vi "AlliGator Create New Empty Phasor Plot.vi"(8 "Error In":errorcluster, 11 "Phasor Graph Ref":refnum<vi>) -> (0 "Error Out":errorcluster, 1 "Plot Name":string, 2 "Plot Array out":cluster{"X Array":dbl[], "Y Array":dbl[]}[](array[cluster]), 3 "Phasor Graph Ref (dup)":refnum<vi>)   [LabVIEW 2021, in "AlliGator Phasor Graph.lvlib"]
doc: "Creates empty plot in the Phasor Graph."
uses:
  <vilib>/Utility/error.llb/Error Cluster From Error Code.vi
  <vilib>/ErrorRing/Error Ring.xnode
  AlliGator Phasor Graph.lvlib
  Graphs/XY Graph/XY Graph Add-Ons.lvlib
panel:
  # "see the AlliGator License on the block diagram (Ctrl+E or Window:Show Block Diagram)"
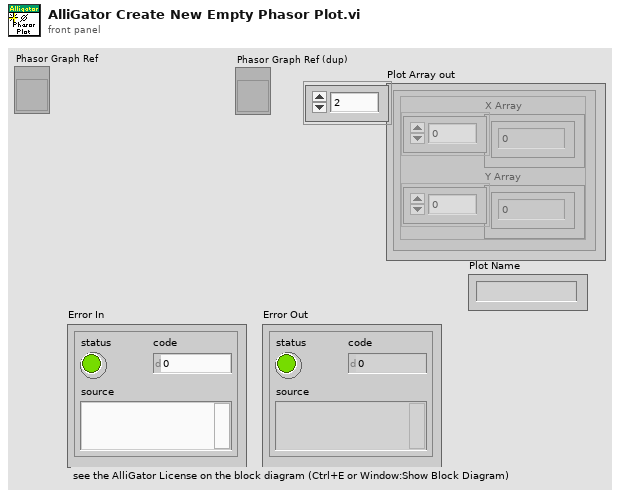
[diagram p1: front panel]
types:
  T1 = typedef "XY Graph Add-Ons.lvlib/XY Graph Refnum.ctl" = refnum<vi>
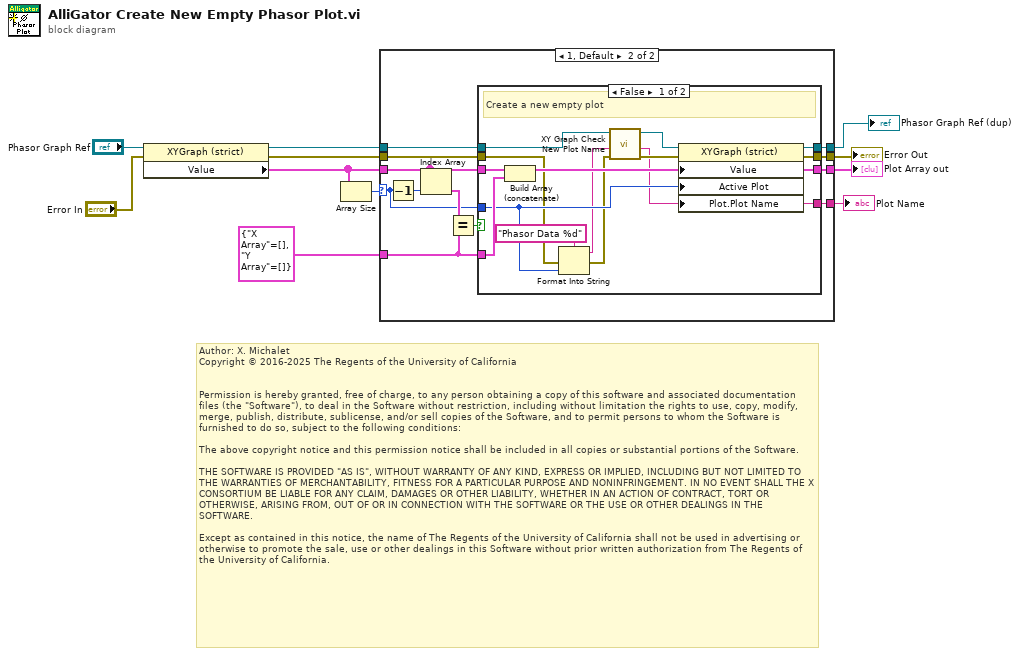
[diagram p0: block diagram]
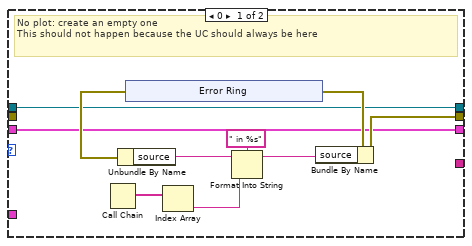
[diagram p2: hidden frame]
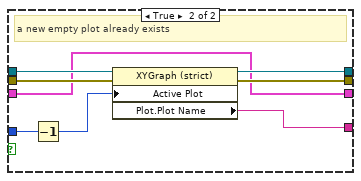
[diagram p3: hidden frame]
diagram:
  # "Author: X. Michalet\nCopyright © 2016-2025 The Regents of the University of California\n \n\nPermission is hereby granted, free of charge, to any person obtaining a copy of this software and associated documentation files (the \"Software\"), to deal in the Software without restriction, including without limitation the rights to use, copy, modify, merge, publish, distribute, sublicense, and/or sell copies of the Software, and to permit persons to whom the Software is furnished to do so, subject to the following conditions:\n\nThe above copyright notice and this permission notice shall be included in all copies or substantial portions of the Software.\n\nTHE SOFTWARE IS PROVIDED \"AS IS\", WITHOUT WARRANTY OF ANY KIND, EXPRESS OR IMPLIED, INCLUDING BUT NOT LIMITED TO THE WARRANTIES OF MERCHANTABILITY, FITNESS FOR A PARTICULAR PURPOSE AND NONINFRINGEMENT. IN NO EVENT SHALL THE X CONSORTIUM BE LIABLE FOR ANY CLAIM, DAMAGES OR OTHER LIABILITY, WHETHER IN AN ACTION OF CONTRACT, TORT OR OTHERWISE, ARISING FROM, OUT OF OR IN CONNECTION WITH THE SOFTWARE OR THE USE OR OTHER DEALINGS IN THE SOFTWARE.\n\nExcept as contained in this notice, the name of The Regents of the University of California shall not be used in advertising or otherwise to promote the sale, use or other dealings in this Software without prior written authorization from The Regents of the University of California."
  n1 = property class="XYGraph (strict)"(reference="Phasor Graph Ref", error in="Error In") -> (reference out=w5:refnum<vi>, error out=w4:errorcluster, "Value"=w7:cluster{"X Array":dbl[], "Y Array":dbl[]}[])
  n2 = Array Size(array=w7) -> (size(s)=w9:i32)
  n3 = case shown="1, Default" w9 {
    selector: w9 -> [_ w27]
    tunnel: cluster{"X Array":dbl[], "Y Array":dbl[]} {"X Array"=[], "Y Array"=[]} ("array") -> [_ w33]
    tunnel: [w12 w36] -> w10
    tunnel: w7 -> [w12 w35]
    tunnel: w5 -> [w13 w31]
    tunnel: w4 -> [_ w30]
    tunnel: [w20 w29] -> w3
    tunnel: [w13 w26] -> w2
    tunnel: [_ w25] -> w1
    frame 0 {
      # "No plot: create an empty one\nThis should not happen because the UC should always be here"
      n4 = Call Chain() -> (call chain=w15:string[])
      n5 = xnode "Error Ring"() -> ("error out"=w19:errorcluster)
      n6 = Unbundle By Name(w19) -> ("source"=w18:string)
      n7 = Index Array(array=w15) -> (element=w14:string)  [unwired: 1 in]
      n8 = Format Into String(format string=" in %s", initial string=w18, w14) -> (resulting string=w17:string)  [unwired: 1 in, 1 out]
      n9 = Bundle By Name(cluster=w19, "source"=w17) -> (w20:errorcluster)
    }
    frame 1, Default {
      n10 = Decrement(x=w27) -> (x-1=w28:i32)
      n11 = Index Array(array=w35, index=w28) -> (element=w34:cluster{"X Array":dbl[], "Y Array":dbl[]})
      n12 = Equal?(x=w34, y=w33) -> (x = y?=w32:bool)
      n13 = case shown="False" w32 {
        tunnel: [w48 w54] -> w36
        tunnel: w35 -> [w50 w54]
        tunnel: w33 -> [w49 _]
        tunnel: w31 -> [w46 w58]
        tunnel: w30 -> [w40 w56]
        tunnel: [w47 w55] -> w29
        tunnel: w27 -> [w42 w53]
        tunnel: [w38 w57] -> w26
        tunnel: [w37 w51] -> w25
        frame False {
          # "Create a new empty plot"
          n14 = Build Array (concatenate)(w50, w49) -> (w48:cluster{"X Array":dbl[], "Y Array":dbl[]}[])
          n15 = Format Into String(format string="Phasor Data %d" ("New Plot Name (in)"), error in=w40, w42) -> (resulting string=w41:string, error out=w39:errorcluster)  [unwired: 1 in]
          n16 = call "XY Graph Check New Plot Name.vi"("Error In"=w39, "New Plot Name (in)"=w41, "Multiplot XY Graph Refnum in"=w46) -> ("Error Out"=w44:errorcluster, "New Plot Name (out)"=w37:string, "Multiplot XY Graph Refnum out"=w45:T1)  [unwired: 6 in]
          n17 = property class="XYGraph (strict)"(reference=w45, error in=w44, "Value"=w48, "Active Plot"=w42, "Plot.Plot Name"=w37) -> (reference out=w38:T1, error out=w47:errorcluster)
        }
        frame True {
          # "a new empty plot already exists"
          n18 = Decrement(x=w53) -> (x-1=w52:i32)
          n19 = property class="XYGraph (strict)"(reference=w58, error in=w56, "Active Plot"=w52) -> (reference out=w57:refnum<vi>, error out=w55:errorcluster, "Plot.Plot Name"=w51:string)
        }
      }
    }
  }
  "Plot Array out" <- w10
  "Error Out" <- w3
  "Phasor Graph Ref (dup)" <- w2
  "Plot Name" <- w1
